vi "Untitled 7.vi"() -> ()   [LabVIEW 2015]
uses:
  <vilib>/NIScanEngine/faults/Fault.ctl
panel:
  out "fault list":T1[](array[typedef]) {"level" items=["Minor Fault", "Major Fault", "Unrecoverable Fault"]}
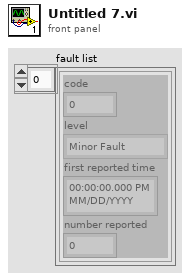
[diagram p1: front panel]
types:
  T1 = typedef "Fault.ctl" = cluster{"code":i32, "level":i32, "first reported time":timestamp, "number reported":u32}
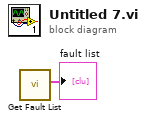
[diagram p0: block diagram]
diagram:
  n1 = call <vilib>:"Get Fault List.vi"() -> ("fault list"=→"fault list":T1[])  [unwired: 10 in, 1 out]
